vi "Que_Valid.vi"(8 "error in (no error)":errorcluster caption="error in", 11 "Queue Name(unamed)":string) -> (0 "error out":errorcluster caption="error Out", 1 "Not Exist?":bool)   [LabVIEW 2016]
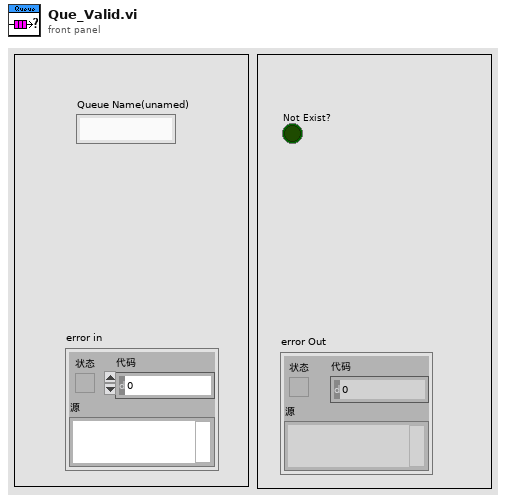
[diagram p1: front panel]
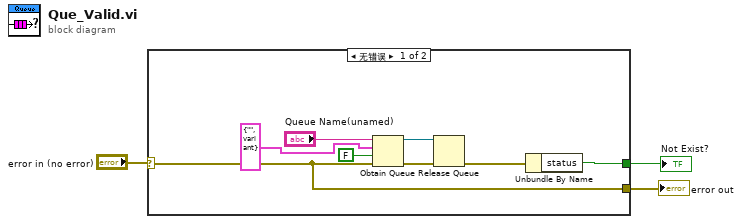
[diagram p0: block diagram]
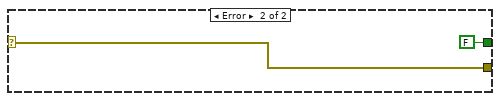
[diagram p2: hidden frame]
diagram:
  n1 = case shown="无错误" "error in (no error)" {
    selector: "error in (no error)" -> [w10 w13]
    tunnel: [w10 w13] -> w2
    tunnel: [w6 FALSE ("status")] -> w1
    frame No Error {
      n2 = Obtain Queue(name (unnamed)="Queue Name(unamed)", element data type=cluster{string, "变体":variant} {"", "变体"=variant} ("DataType"), create if not found? (T)=FALSE ("如未找到是否创建？(T)"), error in (no error)=w10) -> (queue out=w8:refnum<queue>, error out=w9:errorcluster)  [unwired: 1 in, 1 out]
      n3 = Release Queue(queue=w8, error in (no error)=w9) -> (error out=w7:errorcluster)  [unwired: 1 in, 2 out]
      n4 = Unbundle By Name(w7) -> ("status"=w6:bool)
    }
    frame Error {
    }
  }
  "error out" <- w2
  "Not Exist?" <- w1
